vi "SmartSEM Remote API set float.vi"(5 "wait (ms)":u32, 7 "Iterations":u32=3, 8 "error in":errorcluster, 9 "vValue":sgl, 10 "lpszParam":string, 11 "Api":refnum<k7>(container)) -> (0 "error out":errorcluster, 3 "Api out":refnum<k7>)   [LabVIEW 2018]
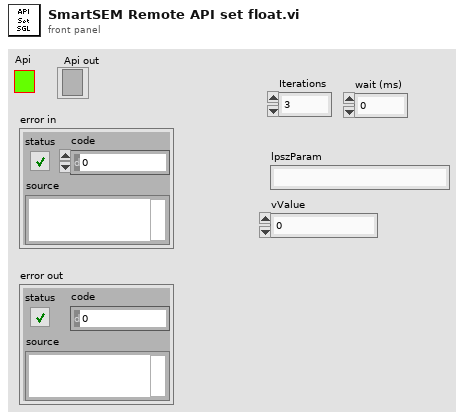
[diagram p1: front panel]
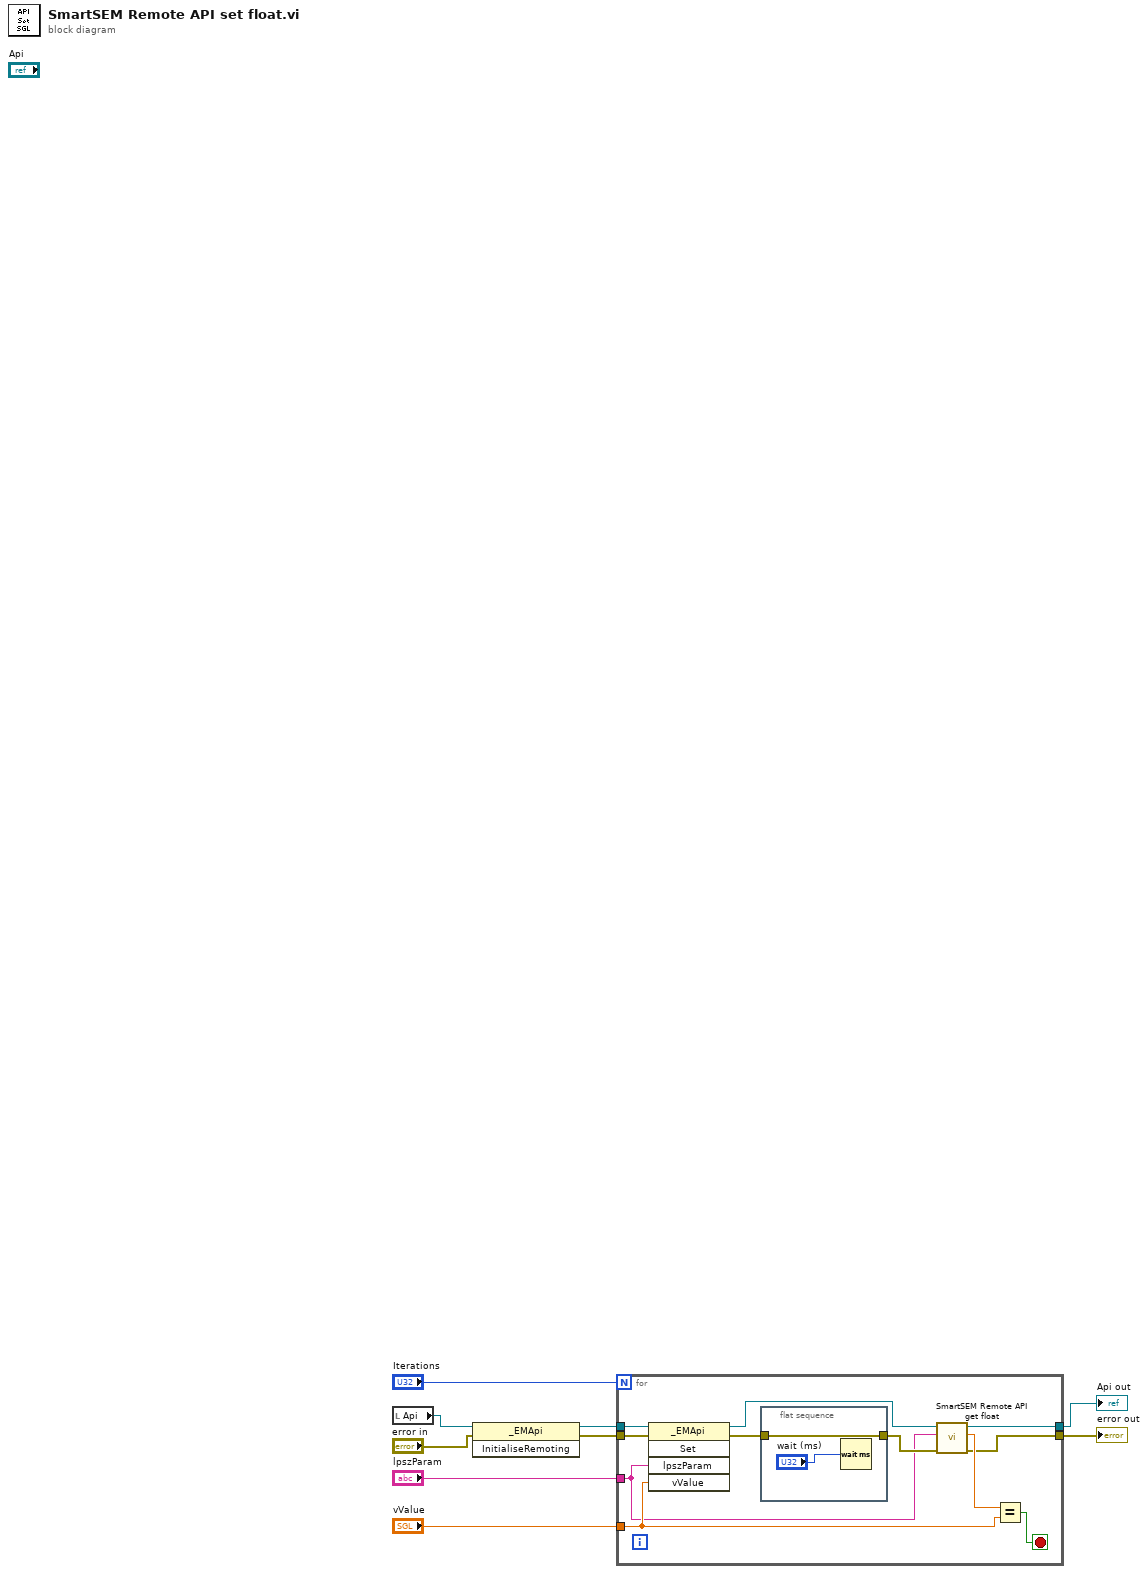
[diagram p0: block diagram]
diagram:
  n1 = local read "Api"() -> (w9:refnum<k7>)
  n2 = invoke class="_EMApi" method="InitialiseRemoting"(reference=w9, error in="error in") -> (reference out=w8:refnum<k7>, error out=w7:errorcluster)  [unwired: 1 in, 1 out]
  n3 = for {
    N: "Iterations" -> [_]
    tunnel: w8 -> [w20]
    tunnel: w7 -> [w19]
    tunnel: [w11] -> w3
    tunnel: [w10] -> w2
    tunnel: "vValue" -> [w17]
    tunnel: "lpszParam" -> [w13]
    stop <- w18 stop-if-true
    n4 = invoke class="_EMApi" method="Set"(reference=w20, error in=w19, "lpszParam"=w13, "vValue"=w17) -> (reference out=w14:refnum<k7>, error out=w16:errorcluster)  [unwired: 1 in, 3 out]
    n5 = flat-sequence {
      tunnel: [w22] -> w15
      tunnel: w16 -> [w22]
      frame #0 {
        n6 = Wait (ms)(milliseconds to wait="wait (ms)") -> ()  [unwired: 1 out]
      }
    }
    n7 = call "SmartSEM Remote API get float.vi"("error in"=w15, "lpszParam"=w13, "Api"=w14) -> ("error out"=w10:errorcluster, "vValue"=w12:sgl, "Api out"=w11:refnum<k7>)  [unwired: 6 in]
    n8 = Equal?(x=w12, y=w17) -> (x = y?=w18:bool)
  }
  "Api out" <- w3
  "error out" <- w2
